vi "数据保存处理.vi"(8 "error in (no error)":errorcluster caption="错误输入（无错误）", 11 "数组":string[](array[string])) -> (0 "error out":errorcluster caption="错误输出", 3 "数组 2":string[](array[string]))   [LabVIEW 2016, in "斯坦道仪器.lvlib"]
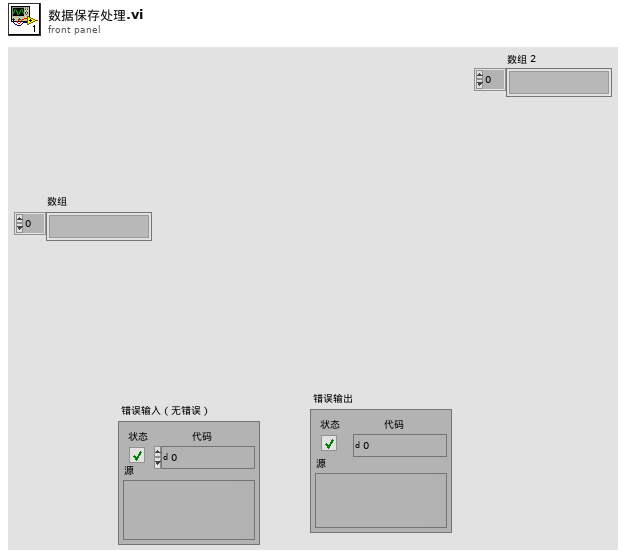
[diagram p1: front panel]
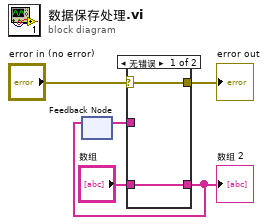
[diagram p0: block diagram]
diagram:
  n1 = feedback #1() -> (w5:string[])  [unwired: 1 in]
  n2 = case shown="无错误" "error in (no error)" {
    selector: "error in (no error)" -> [w6 _]
    tunnel: w5 -> [_ w8]
    tunnel: "数组" -> [w7 _]
    tunnel: [w7 w8] -> w4
    tunnel: [w6 _] -> w1
    frame No Error {
    }
    frame Error {
    }
  }
  "数组 2" <- w4
  "error out" <- w1
  n3 = feedback-in #1(w4) -> ()
